vi "ritartha.vi"() -> ()   [LabVIEW 2020]
uses:
  <instrlib>/Agilent B2900 Series/Public/Configure/Measurement/Configure Measurement (Resistance).vi
  <instrlib>/Agilent B2900 Series/Public/Data/Read Measurement Result (Single Point).vi
  <instrlib>/Agilent B2900 Series/Agilent B2900 Series.lvlib
panel:
  out "error out":errorcluster
  in  "Resistance Range (Ohm)":dbl=2.0
  in  "stop":bool
  out "Waveform Chart":dbl(graph)
  out "Measurement Result":ext
  in  "VISA resource name":refnum<visa-resource-name>="COM1"
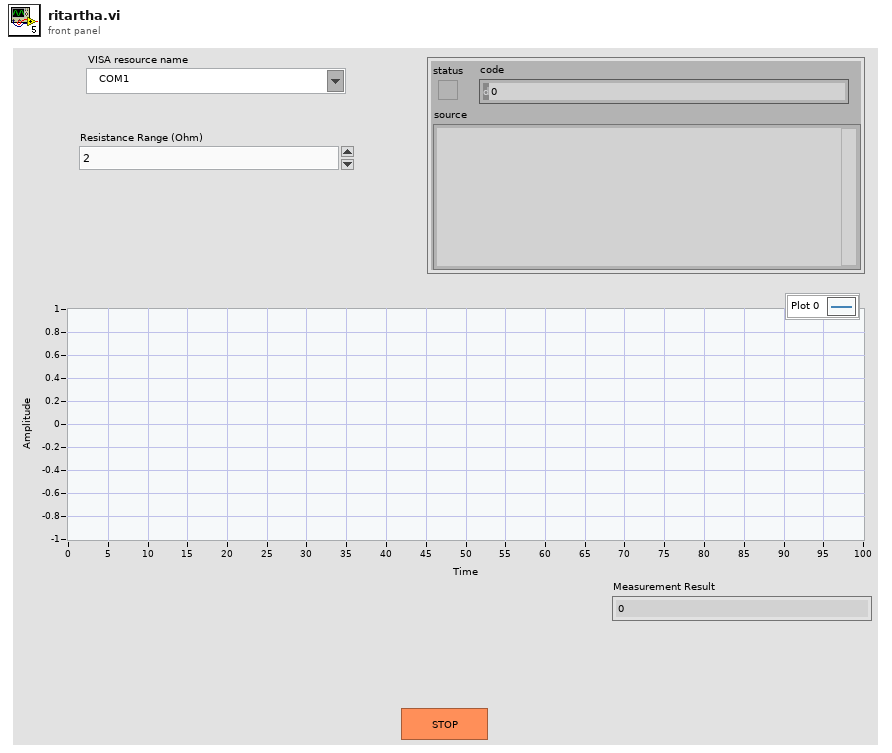
[diagram p1: front panel]
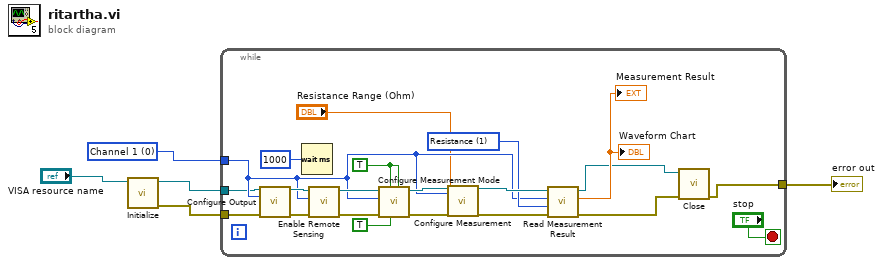
[diagram p0: block diagram]
diagram:
  w5 = 0 items=["Channel 1", "Channel 2"] ("Channel (0: Channel 1)")
  n1 = call <instrlib>:"Initialize.vi"("VISA resource name"="VISA resource name") -> ("error out"=w3:errorcluster, "VISA resource name out"=w2:refnum<visa-resource-name>)  [unwired: 9 in]
  n2 = while {
    tunnel: w5 -> [w14]
    tunnel: w3 -> [w11]
    tunnel: w2 -> [w10]
    tunnel: [w6] -> w1
    stop <- "stop" stop-if-true
    w16 = 1 items=["Current", "Resistance", "Source Output Setting", "Status", "Time", "Voltage"] ("Data Mode (5: Voltage)")
    w17 = TRUE ("Enable Voltage Measurement (T: Enable)")
    n3 = call <instrlib>:"Configure Output.vi"("VISA resource name"=w10, "Channel (0: Channel 1)"=w14, "error in (no error)"=w11) -> ("VISA resource name out"=w22:refnum<visa-resource-name>, "error out"=w26:errorcluster)  [unwired: 11 in]
    n4 = Wait (ms)(milliseconds to wait=u32 1000) -> ()  [unwired: 1 out]
    n5 = call <instrlib>:"Enable Remote Sensing.vi"("error in (no error)"=w26, "Channel (0: Channel 1)"=w14, "VISA resource name"=w22) -> ("error out"=w25:errorcluster, "VISA resource name out"=w21:refnum<visa-resource-name>)  [unwired: 7 in]
    n6 = call <instrlib>:"Configure Measurement Mode.vi"("Enable Current Measurement (T: Enable)"=w17, "Enable Resistance Measurement (F: Disable)"=TRUE, "Enable Voltage Measurement (T: Enable)"=w17, "error in (no error)"=w25, "Channel (0: Channel 1)"=w14, "VISA resource name"=w21) -> ("error out"=w24:errorcluster, "VISA resource name out"=w20:refnum<visa-resource-name>)  [unwired: 4 in]
    n7 = call-poly <instrlib>:"Configure Measurement.vi"("VISA resource name"=w20, "Channel (0: Channel 1)"=w14, "Resistance Range (2 Ohm)"="Resistance Range (Ohm)", "error in (no error)"=w24) -> ("VISA resource name out"=w19:refnum<visa-resource-name>, "error out"=w23:errorcluster)  [unwired: 14 in]
    n8 = call-poly <instrlib>:"Read Measurement Result.vi"("error in (no error)"=w23, "Data Mode (5: Voltage)"=w16, "Channel (0: Channel 1)"=w14, "VISA resource name"=w19) -> ("error out"=w8:errorcluster, "Measurement Result"=→"Measurement Result" →"Waveform Chart":dbl, "VISA resource name out"=w7:refnum<visa-resource-name>)  [unwired: 5 in]
    n9 = call <instrlib>:"Close.vi"("error in (no error)"=w8, "VISA resource name"=w7) -> ("error out"=w6:errorcluster)  [unwired: 9 in]
  }
  "error out" <- w1
